vi "RectangularNode_Create.vi"(0 "reference":refnum<class "RectangularNode.lvclass">, 5 "error in (no error)":errorcluster) -> (14 "reference out":refnum<class "RectangularNode.lvclass">, 19 "error out":errorcluster)   [LabVIEW 2020, in "RectangularNode.lvclass"]
doc: "Creates and initializes a new RectangularNode object.\n\nThis object should be destroyed using a RectangularNode destructor VI or a virtual base class destructor VI.\n\n[GOOP 2.1]"
uses:
  <resource>/Framework/Providers/Open_GDS/UML/RectangularNode_class/RectangularNode.lvclass
  C:/Program Files (x86)/National Instruments/LabVIEW 2020/resource/Framework/Providers/Open_GDS/UML/AbstractNode_class/AbstractNode.lvclass
  <resource>/Framework/Providers/Open_GDS/UML/General/Rectangle/Rectangle Rectangle2D.ctl
  <resource>/Framework/Providers/Open_GDS/UML/AbstractNode_class/AbstractNode.lvclass
panel:
  # "The input reference should only\nbe wired when this method is called\nby a sub class constructor."
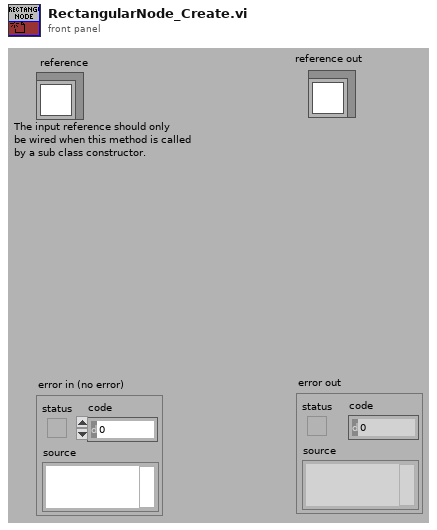
[diagram p1: front panel]
types:
  T1 = typedef "Rectangle Rectangle2D.ctl" = cluster{"x":dbl, "y":dbl, "width":dbl, "height":dbl}
  T2 = typedef "RectangularNode.lvclass/ObjectAttributes.ctl" = cluster{"bounds":T1}
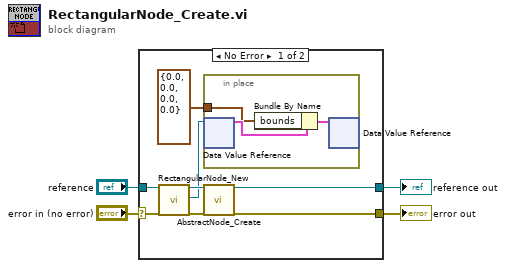
[diagram p0: block diagram]
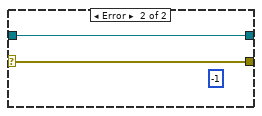
[diagram p2: hidden frame]
diagram:
  n1 = case shown="No Error" "error in (no error)" {
    selector: "error in (no error)" -> [w12 w17]
    tunnel: [w5 w16] -> w4
    tunnel: [w7 w17] -> w3
    tunnel: "reference" -> [w11 w16]
    frame No Error {
      n2 = call <resource>:"RectangularNode_New.vi"("reference in"=w11, "error in (no error)"=w12) -> ("reference out"=w9:refnum<class "RectangularNode.lvclass">, "DVRRefOut"=w6:refnum<data-value>, "error out"=w10:errorcluster)  [unwired: 2 in, 13 out]
      n3 = in-place {
        in-place-border: T1 {"x"=0.0, "y"=0.0, "width"=0.0, "height"=0.0} ("bounds") -> [w14]
        n4 = in-place-dvr #1(w6) -> (w15:T2)  [unwired: 1 out]
        n5 = Bundle By Name(cluster=w15, "bounds"=w14) -> (w13:T2)
        n6 = in-place-dvr #1(w13) -> ()  [unwired: 2 out]
      }
      n7 = call <resource>:"AbstractNode_Create.vi"("reference"=w9, "error in (no error)"=w10) -> ("reference out"=w5:refnum<class "RectangularNode.lvclass">, "error out"=w7:errorcluster)  [unwired: 1 in, 15 out]
    }
    frame Error {
      (unwired) -1 ("Nr of open handles")
    }
  }
  "error out" <- w3
  "reference out" <- w4
